vi "main.vi"() -> ()   [LabVIEW 2019]
uses:
  status_cluster_typedef.ctl
  states_enum_typedef.ctl
  <vilib>/Instr/_visa.llb/VISA Configure Serial Port (Instr).vi
panel:
  out "Status":T1
  in  "Disconnect":bool
  in  "Connect":bool
  in  "VISA resource name":refnum<visa-resource-name>
  in  "Stop":bool
  in  "Send":bool
  in  "Command Prompt":string
  out "Temperature Chart":cluster{"PV":dbl, "SP":dbl}(graph)
  in  "Fans":bool
  in  "Master Power":bool
  in  "Set Point":dbl
  in  "Mode":enum16{"Heat", "Cool", "Standby"}(ring)
  # "Thermal Chamber Controller"
  # "°C"
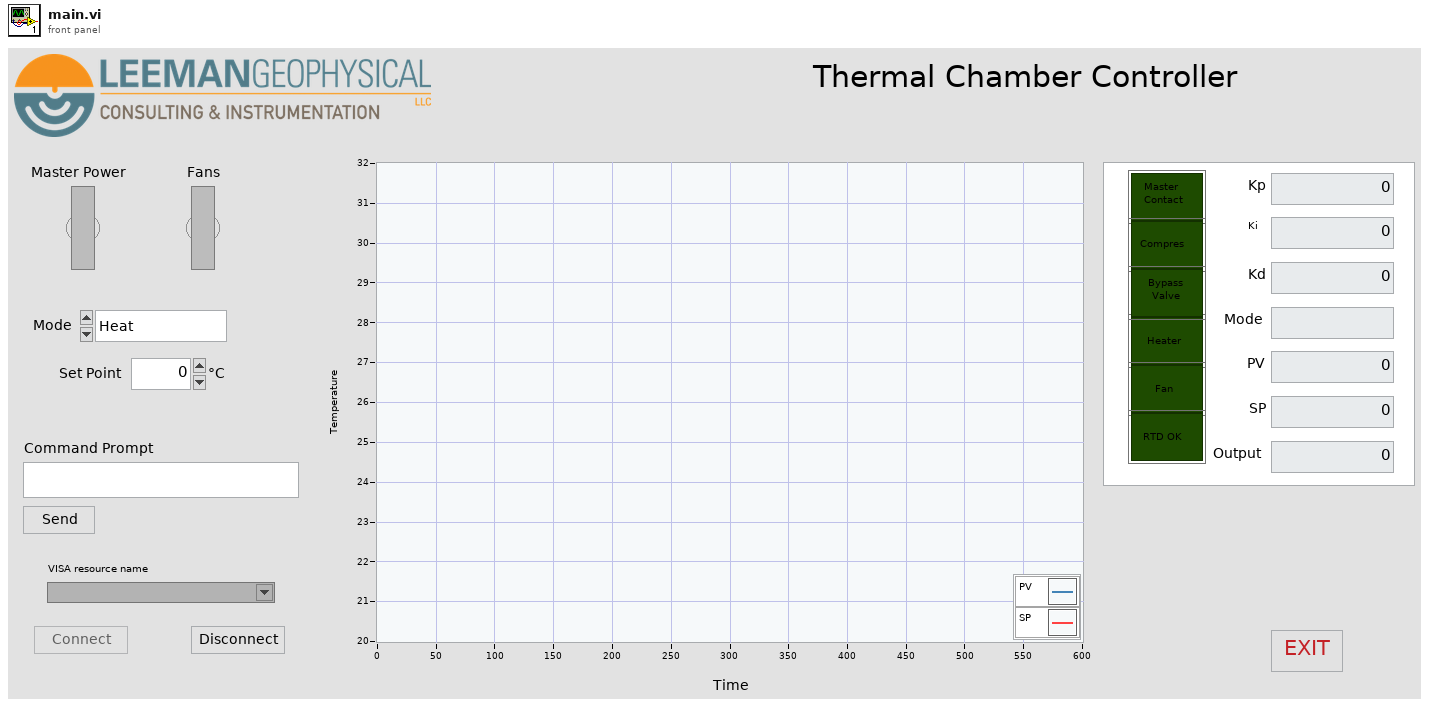
[diagram p1: front panel]
types:
  T1 = typedef "status_cluster_typedef.ctl" = cluster{"Master\nContact":bool, "Heater":bool, "Fan":bool, "Compres":bool, "Bypass\nValve":bool, "Kp":dbl, "Ki":dbl, "Kd":dbl, "Mode":string, "PV":dbl, "SP":dbl, "RTD OK":bool, "Output":dbl}
  T2 = typedef "states_enum_typedef.ctl" = enum16{"ChangePower", "ChangeFan", "ChangeMode", "Shutdown", "Initialize", "Wait", "Disconnect", "Connect", "FansOn", "FansOff", "SetCool", "SetWarm", "SetStandby", "SetTemp", "PowerOn", "PowerOff", "SendCommand", "Read"}
  T3 = enum8{"Enabled", "Disabled", "Disabled and Grayed Out"}
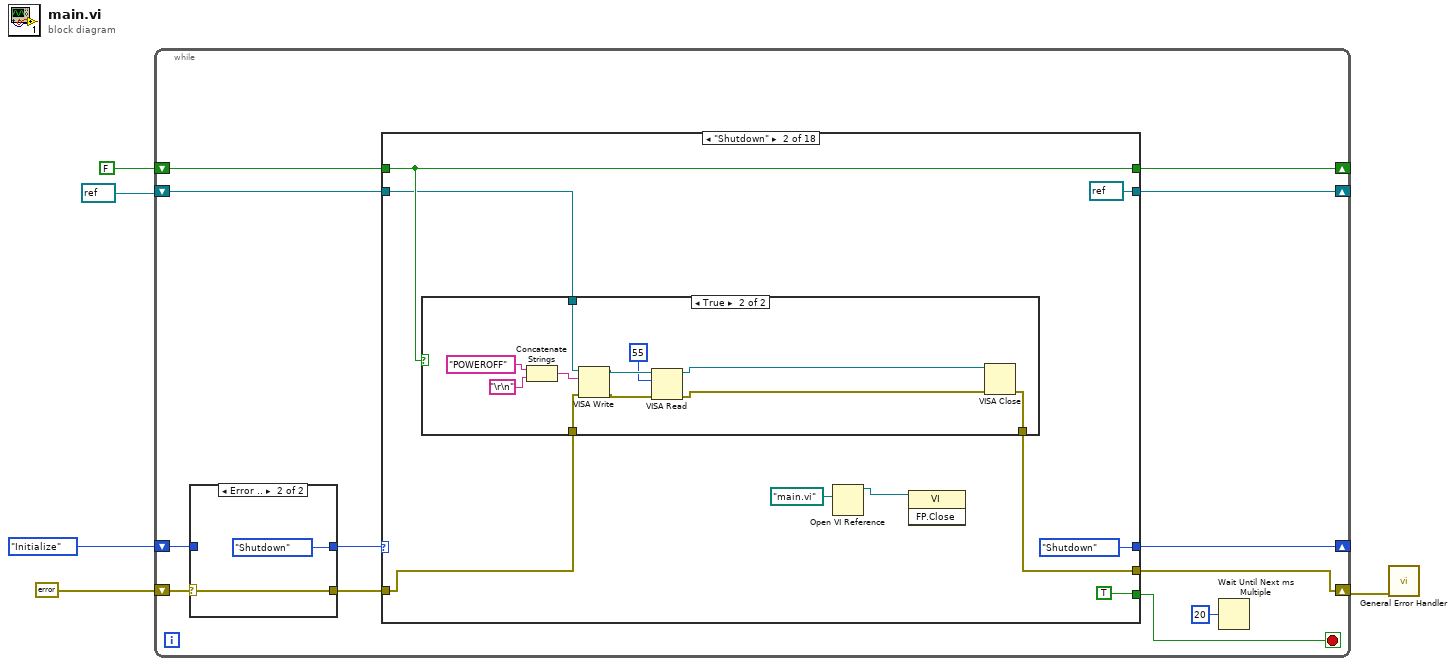
[diagram p0: block diagram]
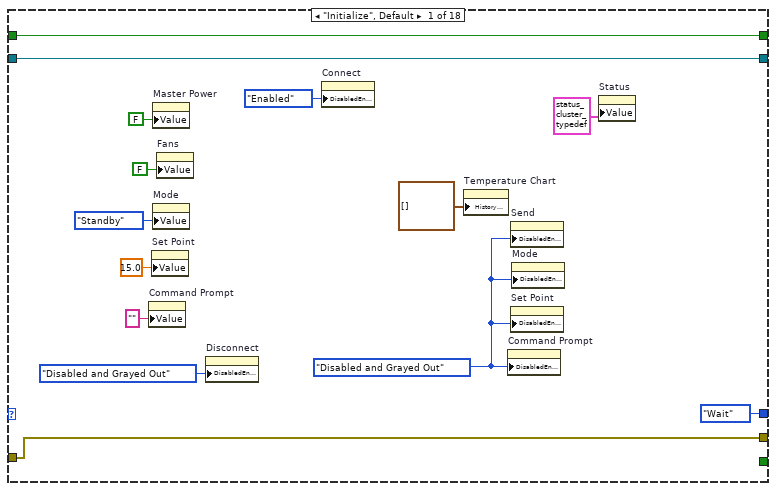
[diagram p3: hidden frame]
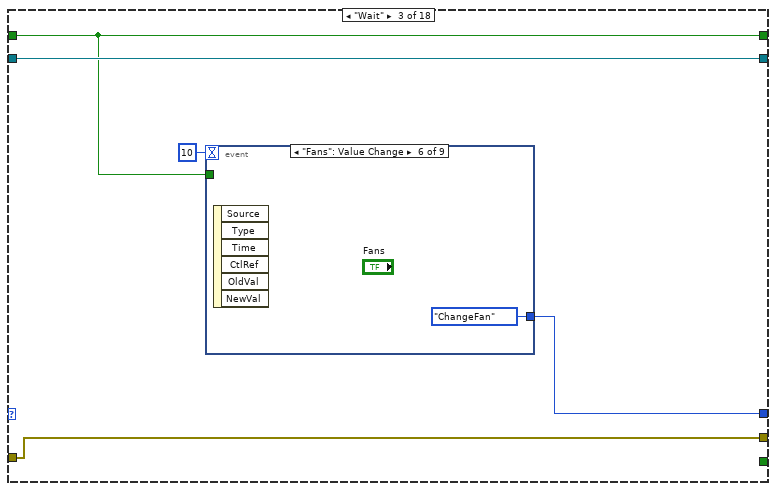
[diagram p5: hidden frame]
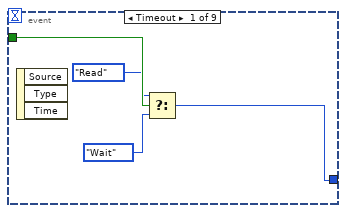
[diagram p6: hidden frame]
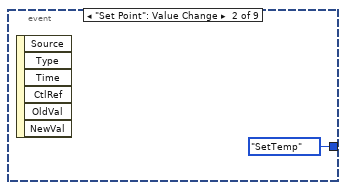
[diagram p7: hidden frame]
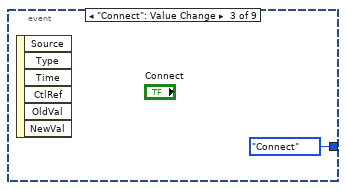
[diagram p8: hidden frame]
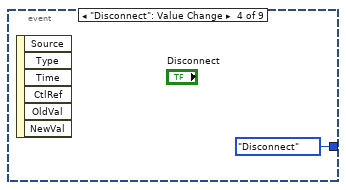
[diagram p9: hidden frame]
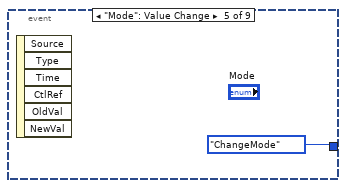
[diagram p10: hidden frame]
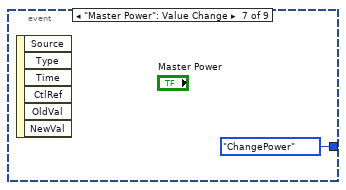
[diagram p11: hidden frame]
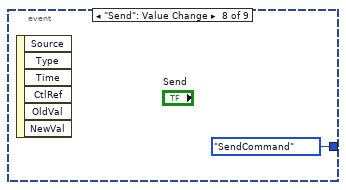
[diagram p12: hidden frame]
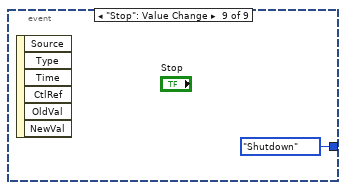
[diagram p13: hidden frame]
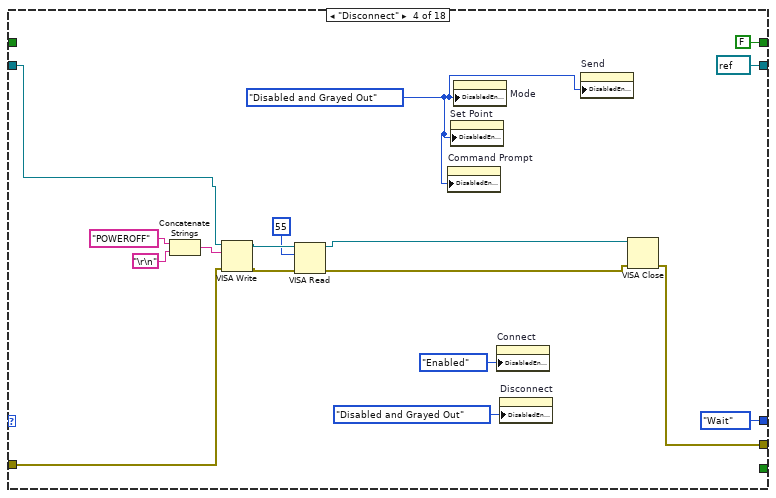
[diagram p14: hidden frame]
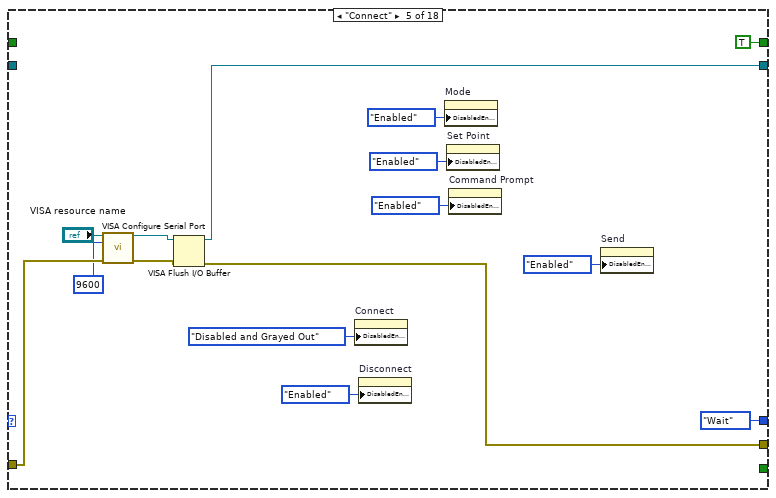
[diagram p15: hidden frame]
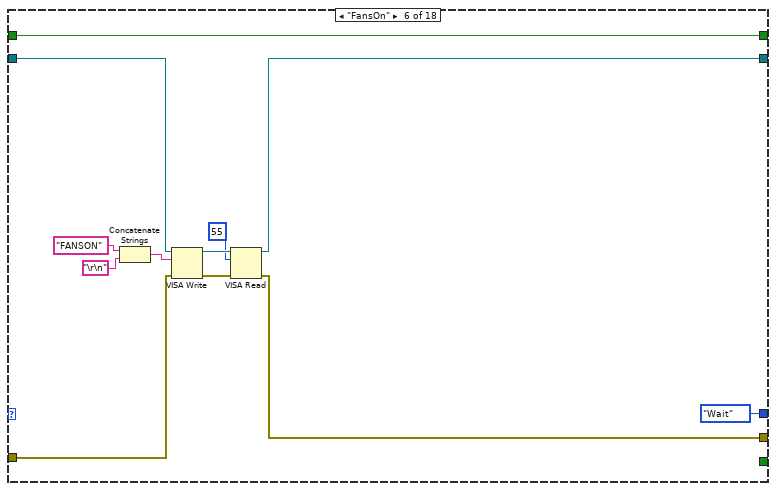
[diagram p16: hidden frame]
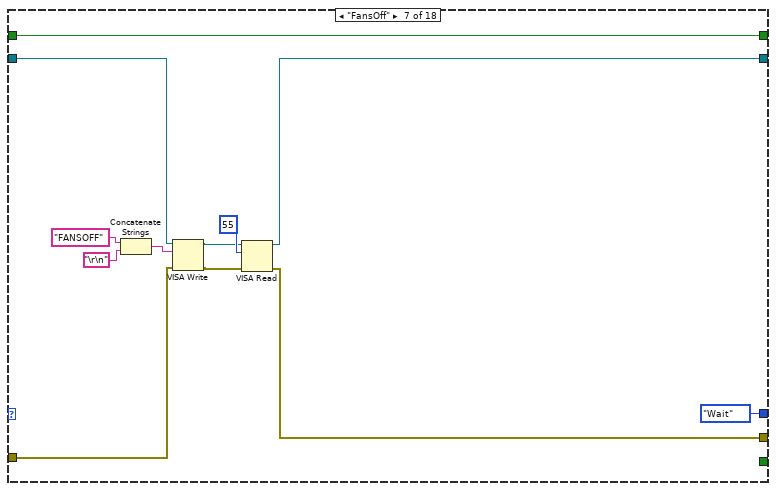
[diagram p17: hidden frame]
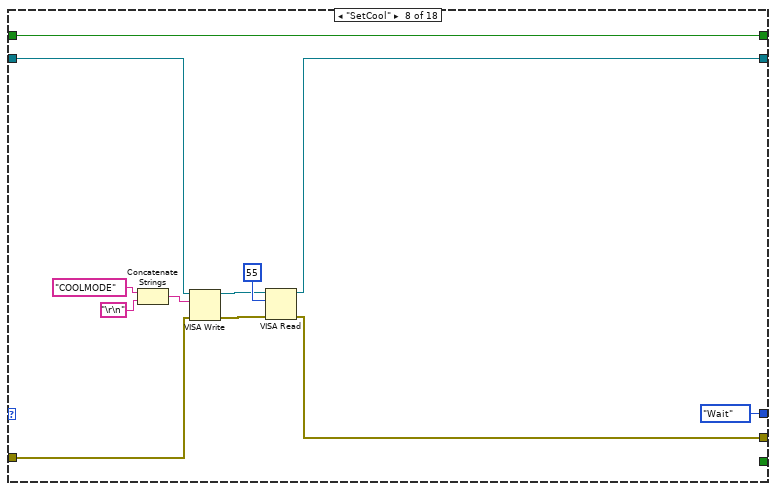
[diagram p18: hidden frame]
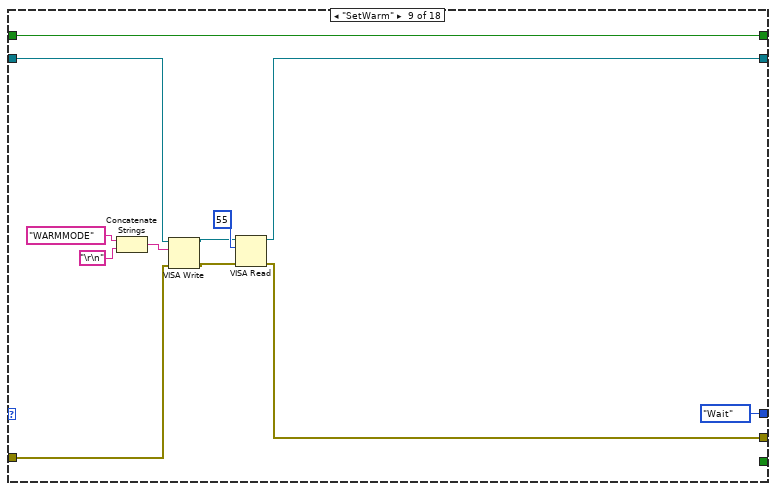
[diagram p19: hidden frame]
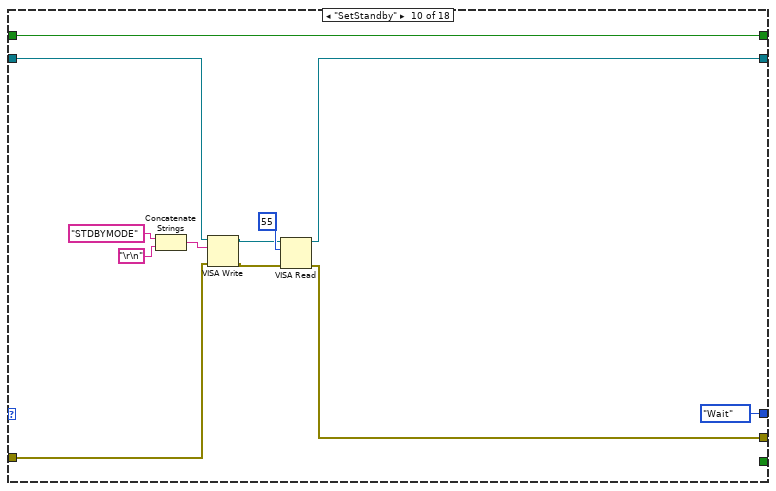
[diagram p20: hidden frame]
diagram:
  n1 = while {
    shift-right: [w13] -> _
    shift-left: states_enum_typedef."Initialize" -> [w17]
    shift-right: [w12] -> w1
    shift-left: errorcluster {"status"=FALSE, "code"=0, "source"=""} ("error constant") -> [w15]
    shift-right: [w9] -> _
    shift-left: FALSE -> [w10]
    shift-right: [w7] -> _
    shift-left: refnum<visa-resource-name> refnum ("VISA resource name") -> [w8]
    stop <- w14 stop-if-true
    n2 = case shown="Error .." w15 {
      selector: w15 -> [w18 w20]
      tunnel: [w19 states_enum_typedef."Shutdown"] -> w16
      tunnel: w17 -> [w19 _]
      tunnel: [w18 w20] -> w11
      frame No Error {
      }
      frame Error {
      }
    }
    n3 = case shown="\"Shutdown\"" w16 {
      tunnel: [_ TRUE _ _ _ _ _ _ _ _ _ _ _ _ _ _ _ _] -> w14
      tunnel: [states_enum_typedef."Wait" states_enum_typedef."Shutdown" w61 states_enum_typedef."Wait" states_enum_typedef."Wait" states_enum_typedef."Wait" states_enum_typedef."Wait" states_enum_typedef."Wait" states_enum_typedef."Wait" states_enum_typedef."Wait" states_enum_typedef."Wait" states_enum_typedef."Wait" states_enum_typedef."Wait" states_enum_typedef."Wait" states_enum_typedef."Wait" w238 w244 w253] -> w13
      tunnel: [w34 w39 w60 w77 w95 w108 w120 w131 w142 w154 w167 w182 w194 w205 w221 w237 w243 w252] -> w12
      tunnel: w11 -> [w34 w40 w60 w78 w104 w113 w125 w136 w147 w160 w171 w187 w199 w212 w223 w237 w243 w252]
      tunnel: w10 -> [w35 w41 w58 _ _ w112 w124 w141 w149 w161 w177 w188 w200 w210 w227 w235 w247 w251]
      tunnel: [w35 w41 w58 FALSE TRUE w112 w124 w141 w149 w161 w177 w188 w200 w210 w227 w235 w247 w251] -> w9
      tunnel: w8 -> [w32 w38 w59 w79 _ w115 w126 w137 w150 w162 w178 w189 w201 w213 w224 w236 w246 w250]
      tunnel: [w32 refnum<visa-resource-name> refnum ("VISA resource name") w59 refnum<visa-resource-name> refnum ("VISA resource name") w96 w107 w121 w130 w143 w155 w168 w181 w193 w206 w222 w236 w246 w250] -> w7
      frame "Initialize", Default {
        w23 = T3."Disabled and Grayed Out" ("Disabled")
        n4 = property on="Command Prompt" class="Str"("Value"="" ("Command Prompt")) -> ()  [unwired: 2 in, 2 out]
        n5 = property on="Set Point" class="DigNum (strict)"("Value"=15.0 ("Set Point")) -> ()  [unwired: 2 in, 2 out]
        n6 = property on="Master Power" class="Bool (strict)"("Value"=FALSE ("Master Power")) -> ()  [unwired: 2 in, 2 out]
        n7 = property on="Mode" class="Enum (strict)"("Value"=enum16{"Heat", "Cool", "Standby"}."Standby" ("Mode")) -> ()  [unwired: 2 in, 2 out]
        n8 = property on="Fans" class="Bool (strict)"("Value"=FALSE ("Fans")) -> ()  [unwired: 2 in, 2 out]
        n9 = property on="Disconnect" class="Bool"("DisabledEnum"=T3."Disabled and Grayed Out" ("Disabled")) -> ()  [unwired: 2 in, 2 out]
        n10 = property on="Connect" class="Bool"("DisabledEnum"=T3."Enabled" ("Disabled")) -> ()  [unwired: 2 in, 2 out]
        n11 = property on="Temperature Chart" class="WFChart (strict)"("History Data"=cluster{"PV":dbl, "SP":dbl}[] []) -> ()  [unwired: 2 in, 2 out]
        n12 = property on="Command Prompt" class="Str"("DisabledEnum"=w23) -> ()  [unwired: 2 in, 2 out]
        n13 = property on="Send" class="Bool"("DisabledEnum"=w23) -> ()  [unwired: 2 in, 2 out]
        n14 = property on="Set Point" class="DigNum (strict)"("DisabledEnum"=w23) -> ()  [unwired: 2 in, 2 out]
        n15 = property on="Mode" class="Enum (strict)"("DisabledEnum"=w23) -> ()  [unwired: 2 in, 2 out]
        n16 = property on="Status" class="Clust (strict)"("Value"=T1 {"Master\nContact"=FALSE, "Heater"=FALSE, "Fan"=FALSE, "Compres"=FALSE, "Bypass\nValve"=FALSE, "Kp"=0.0, "Ki"=0.0, "Kd"=0.0, "Mode"="DISCONN", "PV"=0.0, "SP"=0.0, "RTD OK"=FALSE, "Output"=0.0} ("Status")) -> ()  [unwired: 2 in, 2 out]
      }
      frame "Shutdown" {
        n17 = case shown="True" w41 {
          tunnel: w40 -> [w45 w50]
          tunnel: [w45 w49] -> w39
          tunnel: w38 -> [_ w48]
          frame False {
          }
          frame True {
            n18 = Concatenate Strings("POWEROFF" ("write buffer"), "\r\n") -> (w54:string)
            n19 = VISA Write(VISA resource name=w48, write buffer=w54, error in (no error)=w50) -> (VISA resource name out=w55:refnum<visa-resource-name>, error out=w56:errorcluster)  [unwired: 1 out]
            n20 = VISA Read(VISA resource name=w55, byte count=u32 55, error in (no error)=w56) -> (VISA resource name out=w47:refnum<visa-resource-name>, error out=w46:errorcluster)  [unwired: 2 out]
            n21 = VISA Close(VISA resource name=w47, error in (no error)=w46) -> (error out=w49:errorcluster)
          }
        }
        n22 = Open VI Reference(vi path=path "main.vi") -> (vi reference=w37:refnum<vi>)  [unwired: 5 in, 1 out]
        n23 = invoke class="VI" method="FP.Close"(reference=w37) -> ()  [unwired: 2 in, 3 out]
      }
      frame "Wait" {
        n24 = event shown="[5] \"Fans\": Value Change" {
          selector: _ -> [_ _ _ _ _ _ _ _ _]
          dyn-events: _ -> [_ _ _ _ _ _ _ _ _]
          timeout: 10 -> [_ _ _ _ _ _ _ _ _]
          tunnel: [w62 states_enum_typedef."SetTemp" states_enum_typedef."Connect" states_enum_typedef."Disconnect" states_enum_typedef."ChangeMode" states_enum_typedef."ChangeFan" states_enum_typedef."ChangePower" states_enum_typedef."SendCommand" states_enum_typedef."Shutdown"] -> w61
          tunnel: w58 -> [w65 _ _ _ _ _ _ _ _]
          event Timeout {
            n25 = event-data() -> ()  [unwired: 1 in, 3 out]
            n26 = Select(t=states_enum_typedef."Read", s=w65, f=states_enum_typedef."Wait") -> (s? t:f=w62:T2)
          }
          event "Set Point": Value Change {
            n27 = event-data() -> ()  [unwired: 1 in, 6 out]
          }
          event "Connect": Value Change {
            n28 = event-data() -> ()  [unwired: 1 in, 6 out]
          }
          event "Disconnect": Value Change {
            n29 = event-data() -> ()  [unwired: 1 in, 6 out]
          }
          event "Mode": Value Change {
            n30 = event-data() -> ()  [unwired: 1 in, 6 out]
          }
          event "Fans": Value Change {
            n31 = event-data() -> ()  [unwired: 1 in, 6 out]
          }
          event "Master Power": Value Change {
            n32 = event-data() -> ()  [unwired: 1 in, 6 out]
          }
          event "Send": Value Change {
            n33 = event-data() -> ()  [unwired: 1 in, 6 out]
          }
          event "Stop": Value Change {
            n34 = event-data() -> ()  [unwired: 1 in, 6 out]
          }
        }
      }
      frame "Disconnect" {
        w76 = T3."Disabled and Grayed Out" ("Disabled")
        n35 = Concatenate Strings("POWEROFF" ("write buffer"), "\r\n") -> (w83:string)
        n36 = VISA Write(VISA resource name=w79, write buffer=w83, error in (no error)=w78) -> (VISA resource name out=w84:refnum<visa-resource-name>, error out=w85:errorcluster)  [unwired: 1 out]
        n37 = VISA Read(VISA resource name=w84, byte count=u32 55, error in (no error)=w85) -> (VISA resource name out=w74:refnum<visa-resource-name>, error out=w75:errorcluster)  [unwired: 2 out]
        n38 = property on="Command Prompt" class="Str"("DisabledEnum"=w76) -> ()  [unwired: 2 in, 2 out]
        n39 = property on="Set Point" class="DigNum (strict)"("DisabledEnum"=w76) -> ()  [unwired: 2 in, 2 out]
        n40 = property on="Mode" class="Enum (strict)"("DisabledEnum"=w76) -> ()  [unwired: 2 in, 2 out]
        n41 = property on="Connect" class="Bool"("DisabledEnum"=T3."Enabled" ("Disabled")) -> ()  [unwired: 2 in, 2 out]
        n42 = property on="Disconnect" class="Bool"("DisabledEnum"=T3."Disabled and Grayed Out" ("Disabled")) -> ()  [unwired: 2 in, 2 out]
        n43 = property on="Send" class="Bool"("DisabledEnum"=w76) -> ()  [unwired: 2 in, 2 out]
        n44 = VISA Close(VISA resource name=w74, error in (no error)=w75) -> (error out=w77:errorcluster)
      }
      frame "Connect" {
        n45 = call-poly "VISA Configure Serial Port"("VISA resource name"="VISA resource name", "baud rate (9600)"=u32 9600, "error in (no error)"=w104) -> ("VISA resource name out"=w97:refnum<visa-resource-name>, "error out"=w98:errorcluster)  [unwired: 11 in]
        n46 = VISA Flush I/O Buffer(VISA resource name=w97, error in (no error)=w98) -> (VISA resource name out=w96:refnum<visa-resource-name>, error out=w95:errorcluster)  [unwired: 1 in]
        n47 = property on="Connect" class="Bool"("DisabledEnum"=T3."Disabled and Grayed Out" ("Disabled")) -> ()  [unwired: 2 in, 2 out]
        n48 = property on="Disconnect" class="Bool"("DisabledEnum"=T3."Enabled" ("Disabled")) -> ()  [unwired: 2 in, 2 out]
        n49 = property on="Mode" class="Enum (strict)"("DisabledEnum"=T3."Enabled" ("Disabled")) -> ()  [unwired: 2 in, 2 out]
        n50 = property on="Set Point" class="DigNum (strict)"("DisabledEnum"=T3."Enabled" ("Disabled")) -> ()  [unwired: 2 in, 2 out]
        n51 = property on="Command Prompt" class="Str"("DisabledEnum"=T3."Enabled" ("Disabled")) -> ()  [unwired: 2 in, 2 out]
        n52 = property on="Send" class="Bool"("DisabledEnum"=T3."Enabled" ("Disabled")) -> ()  [unwired: 2 in, 2 out]
      }
      frame "FansOn" {
        n53 = Concatenate Strings("FANSON" ("write buffer"), "\r\n") -> (w114:string)
        n54 = VISA Write(VISA resource name=w115, write buffer=w114, error in (no error)=w113) -> (VISA resource name out=w110:refnum<visa-resource-name>, error out=w109:errorcluster)  [unwired: 1 out]
        n55 = VISA Read(VISA resource name=w110, byte count=u32 55, error in (no error)=w109) -> (VISA resource name out=w107:refnum<visa-resource-name>, error out=w108:errorcluster)  [unwired: 2 out]
      }
      frame "FansOff" {
        n56 = Concatenate Strings("FANSOFF" ("write buffer"), "\r\n") -> (w129:string)
        n57 = VISA Write(VISA resource name=w126, write buffer=w129, error in (no error)=w125) -> (VISA resource name out=w119:refnum<visa-resource-name>, error out=w118:errorcluster)  [unwired: 1 out]
        n58 = VISA Read(VISA resource name=w119, byte count=u32 55, error in (no error)=w118) -> (VISA resource name out=w121:refnum<visa-resource-name>, error out=w120:errorcluster)  [unwired: 2 out]
      }
      frame "SetCool" {
        n59 = Concatenate Strings("COOLMODE" ("write buffer"), "\r\n") -> (w140:string)
        n60 = VISA Write(VISA resource name=w137, write buffer=w140, error in (no error)=w136) -> (VISA resource name out=w133:refnum<visa-resource-name>, error out=w132:errorcluster)  [unwired: 1 out]
        n61 = VISA Read(VISA resource name=w133, byte count=u32 55, error in (no error)=w132) -> (VISA resource name out=w130:refnum<visa-resource-name>, error out=w131:errorcluster)  [unwired: 2 out]
      }
      frame "SetWarm" {
        n62 = Concatenate Strings("WARMMODE" ("write buffer"), "\r\n") -> (w153:string)
        n63 = VISA Write(VISA resource name=w150, write buffer=w153, error in (no error)=w147) -> (VISA resource name out=w145:refnum<visa-resource-name>, error out=w144:errorcluster)  [unwired: 1 out]
        n64 = VISA Read(VISA resource name=w145, byte count=u32 55, error in (no error)=w144) -> (VISA resource name out=w143:refnum<visa-resource-name>, error out=w142:errorcluster)  [unwired: 2 out]
      }
      frame "SetStandby" {
        n65 = Concatenate Strings("STDBYMODE" ("write buffer"), "\r\n") -> (w165:string)
        n66 = VISA Write(VISA resource name=w162, write buffer=w165, error in (no error)=w160) -> (VISA resource name out=w157:refnum<visa-resource-name>, error out=w156:errorcluster)  [unwired: 1 out]
        n67 = VISA Read(VISA resource name=w157, byte count=u32 55, error in (no error)=w156) -> (VISA resource name out=w155:refnum<visa-resource-name>, error out=w154:errorcluster)  [unwired: 2 out]
      }
      frame "SetTemp" {
        n68 = Format Value(format string="%.2f", value (0)="Set Point") -> (output string=w172:string)  [unwired: 1 in]
        n69 = Concatenate Strings("SETTEMP " ("write buffer"), w172, "\r\n") -> (w180:string)
        n70 = VISA Write(VISA resource name=w178, write buffer=w180, error in (no error)=w171) -> (VISA resource name out=w169:refnum<visa-resource-name>, error out=w170:errorcluster)  [unwired: 1 out]
        n71 = VISA Read(VISA resource name=w169, byte count=u32 55, error in (no error)=w170) -> (VISA resource name out=w168:refnum<visa-resource-name>, error out=w167:errorcluster)  [unwired: 2 out]
      }
      frame "PowerOn" {
        n72 = Concatenate Strings("POWERON" ("write buffer"), "\r\n") -> (w192:string)
        n73 = VISA Write(VISA resource name=w189, write buffer=w192, error in (no error)=w187) -> (VISA resource name out=w184:refnum<visa-resource-name>, error out=w183:errorcluster)  [unwired: 1 out]
        n74 = VISA Read(VISA resource name=w184, byte count=u32 55, error in (no error)=w183) -> (VISA resource name out=w181:refnum<visa-resource-name>, error out=w182:errorcluster)  [unwired: 2 out]
      }
      frame "PowerOff" {
        n75 = Concatenate Strings("POWEROFF" ("write buffer"), "\r\n") -> (w204:string)
        n76 = VISA Write(VISA resource name=w201, write buffer=w204, error in (no error)=w199) -> (VISA resource name out=w196:refnum<visa-resource-name>, error out=w195:errorcluster)  [unwired: 1 out]
        n77 = VISA Read(VISA resource name=w196, byte count=u32 55, error in (no error)=w195) -> (VISA resource name out=w193:refnum<visa-resource-name>, error out=w194:errorcluster)  [unwired: 2 out]
      }
      frame "SendCommand" {
        n78 = Concatenate Strings("Command Prompt", "\r\n") -> (w216:string)
        n79 = VISA Write(VISA resource name=w213, write buffer=w216, error in (no error)=w212) -> (VISA resource name out=w208:refnum<visa-resource-name>, error out=w207:errorcluster)  [unwired: 1 out]
        n80 = VISA Read(VISA resource name=w208, byte count=u32 55, error in (no error)=w207) -> (VISA resource name out=w206:refnum<visa-resource-name>, error out=w205:errorcluster)  [unwired: 2 out]
      }
      frame "Read" {
        n81 = VISA Read(VISA resource name=w224, byte count=u32 255, error in (no error)=w223) -> (VISA resource name out=w222:refnum<visa-resource-name>, read buffer=w217:string, error out=w221:errorcluster)  [unwired: 1 out]
        n82 = Search/Split String(string=w217, search string/char (-)="\t") -> (offset of match=w220:i32)  [unwired: 1 in, 2 out]
        n83 = Greater Than 0?(x=w220) -> (x > 0?=w219:bool)
        n84 = case shown="True" w219 {
          tunnel: w217 -> [_ w230]
          frame False {
          }
          frame True {
            n85 = call "parse_return_serial.vi"("string"=w230) -> ("Status"=w234:T1)  [unwired: 10 in]
            "Status" <- w234
            n86 = Unbundle By Name(w234) -> ("PV"=w233:dbl, "SP"=w232:dbl, "Master\nContact"=w229:bool, "Fan"=w228:bool)
            n87 = property on="Master Power" class="Bool (strict)"("Value"=w229) -> ()  [unwired: 2 in, 2 out]
            n88 = property on="Fans" class="Bool (strict)"("Value"=w228) -> ()  [unwired: 2 in, 2 out]
            n89 = Bundle("PV"=w233, "SP"=w232) -> (→"Temperature Chart":cluster{"PV":dbl, "SP":dbl})  [unwired: 1 in]
          }
        }
      }
      frame "ChangeMode" {
        n90 = property on="Mode" class="Enum (strict)"() -> ("Value"=w239:enum16{"Heat", "Cool", "Standby"})  [unwired: 2 in, 2 out]
        n91 = case shown="\"Standby\", Default" w239 {
          tunnel: [states_enum_typedef."SetWarm" states_enum_typedef."SetCool" states_enum_typedef."SetStandby"] -> w238
          frame "Heat" {
          }
          frame "Cool" {
          }
          frame "Standby", Default {
          }
        }
      }
      frame "ChangeFan" {
        n92 = property on="Fans" class="Bool (strict)"() -> ("Value"=w245:bool)  [unwired: 2 in, 2 out]
        n93 = case shown="False" w245 {
          tunnel: [states_enum_typedef."FansOff" states_enum_typedef."FansOn"] -> w244
          frame False {
          }
          frame True {
          }
        }
      }
      frame "ChangePower" {
        n94 = property on="Master Power" class="Bool (strict)"() -> ("Value"=w254:bool)  [unwired: 2 in, 2 out]
        n95 = case shown="False" w254 {
          tunnel: [states_enum_typedef."PowerOff" states_enum_typedef."PowerOn"] -> w253
          frame False {
          }
          frame True {
          }
        }
      }
    }
    n96 = Wait Until Next ms Multiple(millisecond multiple=u32 20) -> ()  [unwired: 1 out]
  }
  n97 = call <vilib>:"General Error Handler.vi"("error in (no error)"=w1) -> ()  [unwired: 10 in, 5 out]
